vi "Relay Control.vi"(0 "GEA2 Reference In":refnum<k24>, 5 "Relay":enum16{"Motor Enable", "Valve", "Both"}(ring), 7 "State":enum16{"On", "Off"}(ring), 11 "Error In":errorcluster) -> (4 "GEA2 Reference Out":refnum<k24>, 6 "Pass/Fail?":bool, 8 "Report Text":string, 15 "Error Out":errorcluster)   [LabVIEW 2016, in "Centauro.lvlib"]
doc: "Use this VI to control the state of the motor enable and valve relay."
uses:
  Projects/Centauro.lvlib
  Q:/Common/DLLs/GEA3/GeaCommunication.dll
  Common/DLLs/GEA3/GeaCommunication.dll
  Common/LabVIEW GEA2 Toolkit/LabVIEW_GEA2_Toolkit.lvlibp/type defs/Source_Destination.ctl
  Common/LabVIEW GEA2 Toolkit/LabVIEW_GEA2_Toolkit.lvlibp/type defs/ERD Read Data In.ctl
  Common/LabVIEW GEA2 Toolkit/LabVIEW_GEA2_Toolkit.lvlibp/type defs/Data Type.ctl
  Common/LabVIEW GEA2 Toolkit/LabVIEW_GEA2_Toolkit.lvlibp/type defs/ERD Write Data In.ctl
  Common/LabVIEW GEA2 Toolkit/LabVIEW_GEA2_Toolkit.lvlibp
panel:
  in  "Standalone?":bool
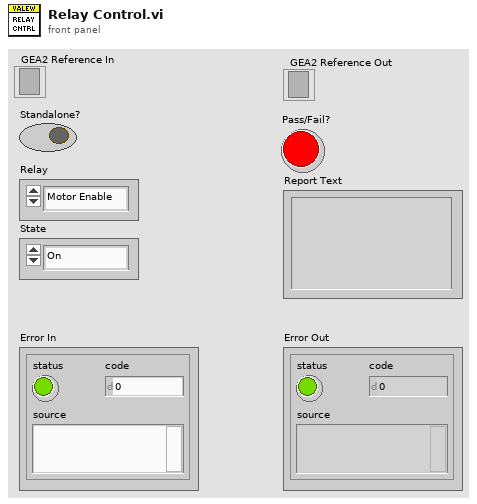
[diagram p1: front panel]
types:
  T1 = typedef "LabVIEW_GEA2_Toolkit.lvlibp/Source_Destination.ctl" = cluster{"Source":u8, "Destination":u8}
  T2 = typedef "LabVIEW_GEA2_Toolkit.lvlibp/ERD Write Data In.ctl" = cluster{"ERD Number":u16, "Data Type":T3, "Data":string}
  T3 = typedef "LabVIEW_GEA2_Toolkit.lvlibp/Data Type.ctl" = enum16{"string", "boolean", "uint8_t", "uint16_t", "uint32_t", "uint64_t", "int8_t", "int16_t", "int32_t", "int64_t"}
  T4 = typedef "LabVIEW_GEA2_Toolkit.lvlibp/ERD Read Data In.ctl" = cluster{"ERD Number":u16, "Data Type":T3}
  T5 = typedef "LabVIEW_GEA2_Toolkit.lvlibp/ERD Read Data Out.ctl" = cluster{"ERD Number":u16, "Data":string}
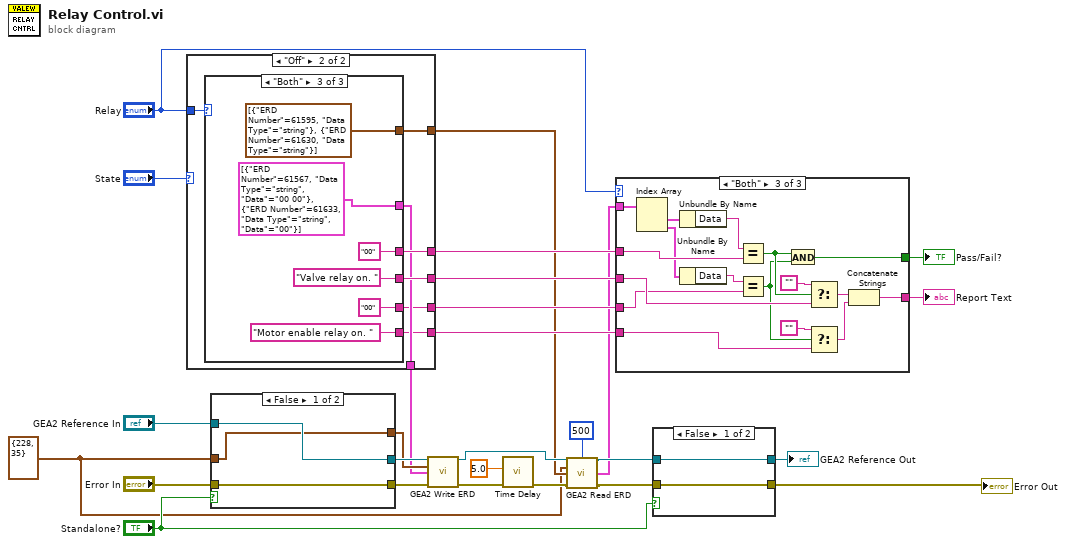
[diagram p0: block diagram]
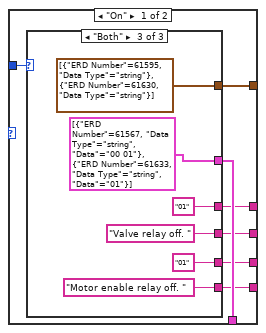
[diagram p2: hidden frame]
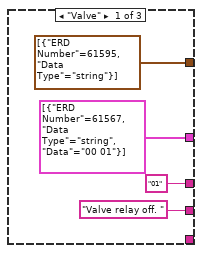
[diagram p3: hidden frame]
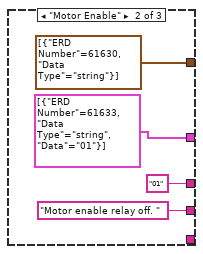
[diagram p4: hidden frame]
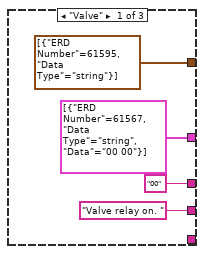
[diagram p5: hidden frame]
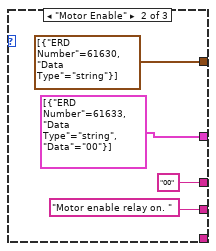
[diagram p6: hidden frame]
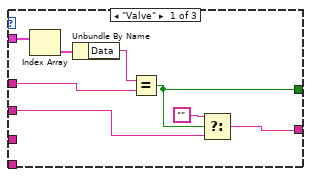
[diagram p7: hidden frame]
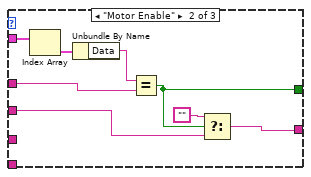
[diagram p8: hidden frame]
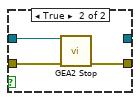
[diagram p9: hidden frame]
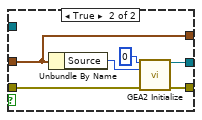
[diagram p10: hidden frame]
diagram:
  w5 = T1 {"Source"=228, "Destination"=35} ("GEA Inputs")
  n1 = case shown="\"Off\"" "State" {
    tunnel: [w34 w52] -> w3
    tunnel: [w33 w54] -> w21
    tunnel: [w32 w53] -> w20
    tunnel: [w31 w55] -> w6
    tunnel: "Relay" -> [w30 w51]
    tunnel: [w28 w50] -> w17
    tunnel: [w29 w49] -> w16
    frame "On" {
      n2 = case shown="\"Both\"" w30 {
        tunnel: [T2[] [{"ERD Number"=61567, "Data Type"=enum."string", "Data"="00 01"}] ("Write ERD List") T2[] [{"ERD Number"=61633, "Data Type"=enum."string", "Data"="01"}] ("Write ERD List") T2[] [{"ERD Number"=61567, "Data Type"=enum."string", "Data"="00 01"}, {"ERD Number"=61633, "Data Type"=enum."string", "Data"="01"}] ("Write ERD List")] -> w34
        tunnel: ["01" ("y") "01" ("y") "01" ("y")] -> w33
        tunnel: ["Valve relay off. " ("f") "Motor enable relay off. " ("f") "Valve relay off. " ("f")] -> w32
        tunnel: [T4[] [{"ERD Number"=61595, "Data Type"=enum."string"}] ("Read ERD List") T4[] [{"ERD Number"=61630, "Data Type"=enum."string"}] ("Read ERD List") T4[] [{"ERD Number"=61595, "Data Type"=enum."string"}, {"ERD Number"=61630, "Data Type"=enum."string"}] ("Read ERD List")] -> w31
        tunnel: [_ _ "01" ("y")] -> w29
        tunnel: [_ _ "Motor enable relay off. " ("f")] -> w28
        frame "Valve" {
        }
        frame "Motor Enable" {
        }
        frame "Both" {
        }
      }
    }
    frame "Off" {
      n3 = case shown="\"Both\"" w51 {
        tunnel: [T2[] [{"ERD Number"=61567, "Data Type"=enum."string", "Data"="00 00"}] ("Write ERD List") T2[] [{"ERD Number"=61633, "Data Type"=enum."string", "Data"="00"}] ("Write ERD List") T2[] [{"ERD Number"=61567, "Data Type"=enum."string", "Data"="00 00"}, {"ERD Number"=61633, "Data Type"=enum."string", "Data"="00"}] ("Write ERD List")] -> w52
        tunnel: ["00" ("y") "00" ("y") "00" ("y")] -> w54
        tunnel: ["Valve relay on. " ("f") "Motor enable relay on. " ("f") "Valve relay on. " ("f")] -> w53
        tunnel: [T4[] [{"ERD Number"=61595, "Data Type"=enum."string"}] ("Read ERD List") T4[] [{"ERD Number"=61630, "Data Type"=enum."string"}] ("Read ERD List") T4[] [{"ERD Number"=61595, "Data Type"=enum."string"}, {"ERD Number"=61630, "Data Type"=enum."string"}] ("Read ERD List")] -> w55
        tunnel: [_ _ "Motor enable relay on. " ("f")] -> w50
        tunnel: [_ _ "00" ("y")] -> w49
        frame "Valve" {
        }
        frame "Motor Enable" {
        }
        frame "Both" {
        }
      }
    }
  }
  n4 = case shown="False" "Standalone?" {
    tunnel: "Error In" -> [w71 w76]
    tunnel: [w71 w74] -> w13
    tunnel: "GEA2 Reference In" -> [w72 _]
    tunnel: [w72 w75] -> w14
    tunnel: w5 -> [w70 w73]
    tunnel: [w70 w73] -> w4
    frame False {
    }
    frame True {
      n5 = Unbundle By Name(w73) -> ("Source"=w77:u8)
      n6 = call "GEA2 Initialize.vi"("Board Index"=0, "Source Address"=w77, "error in"=w76) -> ("GEA2 Reference Out"=w75:refnum<k24>, "error out"=w74:errorcluster)  [unwired: 10 in, 1 out]
    }
  }
  n7 = call "GEA2 Write ERD.vi"("GEA2 Reference In"=w14, "GEA Inputs"=w4, "Write ERD List"=w3, "Error In"=w13) -> ("GEA2 Reference Out"=w11:refnum<k24>, "Error Out"=w9:errorcluster)  [unwired: 9 in, 1 out]
  n8 = call "Time Delay"("error in (no error)"=w9, "Delay Time (s)"=5.0) -> ("error out"=w10:errorcluster)  [unwired: 9 in]
  n9 = call "GEA2 Read ERD.vi"("GEA2 Reference In"=w11, "Read Timeout (ms)"=u32 500, "GEA Inputs"=w5, "Read ERD List"=w6, "Error In"=w10) -> ("GEA2 Reference Out"=w12:refnum<k24>, "ERD Data Out"=w8:T5[], "Error Out"=w7:errorcluster)  [unwired: 7 in, 1 out]
  n10 = case shown="\"Both\"" "Relay" {
    tunnel: [w85 w93 w97] -> w23
    tunnel: w8 -> [w84 w92 w110]
    tunnel: [w81 w89 w98] -> w22
    tunnel: w21 -> [w80 w87 w107]
    tunnel: w20 -> [w79 w88 w106]
    tunnel: w17 -> [_ _ w102]
    tunnel: w16 -> [_ _ w101]
    frame "Valve" {
      n11 = Index Array(array=w84) -> (element=w83:T5)  [unwired: 1 in]
      n12 = Unbundle By Name(w83) -> ("Data"=w82:string)
      n13 = Equal?(x=w82, y=w80) -> (x = y?=w81:bool)
      n14 = Select(t="", s=w81, f=w79) -> (s? t:f=w85:string)
    }
    frame "Motor Enable" {
      n15 = Index Array(array=w92) -> (element=w91:T5)  [unwired: 1 in]
      n16 = Unbundle By Name(w91) -> ("Data"=w90:string)
      n17 = Equal?(x=w90, y=w87) -> (x = y?=w89:bool)
      n18 = Select(t="", s=w89, f=w88) -> (s? t:f=w93:string)
    }
    frame "Both" {
      n19 = Index Array(array=w110) -> (element #1=w109:T5, element #2=w104:T5)  [unwired: 2 in]
      n20 = Unbundle By Name(w109) -> ("Data"=w108:string)
      n21 = Unbundle By Name(w104) -> ("Data"=w105:string)
      n22 = Equal?(x=w108, y=w107) -> (x = y?=w100:bool)
      n23 = Equal?(x=w105, y=w101) -> (x = y?=w99:bool)
      n24 = And(x=w100, y=w99) -> (x .and. y?=w98:bool)
      n25 = Select(t="", s=w100, f=w106) -> (s? t:f=w96:string)
      n26 = Select(t="", s=w99, f=w102) -> (s? t:f=w95:string)
      n27 = Concatenate Strings(w96, w95) -> (w97:string)
    }
  }
  "Pass/Fail?" <- w22
  "Report Text" <- w23
  n28 = case shown="False" "Standalone?" {
    tunnel: w7 -> [w113 w114]
    tunnel: [w113 w115] -> w2
    tunnel: [w112 _] -> w27
    tunnel: w12 -> [w112 w116]
    frame False {
    }
    frame True {
      n29 = call "GEA2 Stop.vi"("GEA2 Reference In"=w116, "Error In"=w114) -> ("Error Out"=w115:errorcluster)  [unwired: 13 in]
    }
  }
  "Error Out" <- w2
  "GEA2 Reference Out" <- w27
